vi "Set_Osc_Conf.vi"(0 "VISA resource name":refnum<visa-resource-name>="Oscilloscope", 1 "Amplitude IN":dbl=0.25, 2 "Trigger Level IN":dbl=0.025, 3 "Pulse Width in seconds IN":dbl=2.5e-09, 5 "error in (no error)":errorcluster, 6 "Channel 1":bool=TRUE, 7 "Channel 3":bool=TRUE, 8 "Channel 2":bool, 9 "Channel 4":bool=TRUE) -> (14 "VISA resource name out":refnum<visa-resource-name>="Oscilloscope", 19 "error out":errorcluster)   [LabVIEW 2012]
uses:
  C/Program Files/National Instruments/LabVIEW 2012/instr.lib/Agilent 8000 Series/Public/Configure/Configure Trigger (Edge).vi
  C/Program Files/National Instruments/LabVIEW 2012/instr.lib/Agilent 8000 Series/Agilent 8000 Series.lvlib
panel:
  in  "Channel 4":i32(ring)=4 items=["Channel 1"=1, "Channel 2"=2, "Channel 3"=3, "Channel 4"=4]
  in  "Vertical Coupling 4":i32(ring)=1 items=["AC", "DC"]
  in  "Probe Attenuation 4":dbl=1.0
  in  "Vertical Range Scaler 4":dbl=1.0
  in  "Vertical Offset 4":dbl
  in  "Input Impedance 4":u32(ring) items=["50 ohms", "1 Mohms"]
  in  "Channel 3":i32(ring)=3 items=["Channel 1"=1, "Channel 2"=2, "Channel 3"=3, "Channel 4"=4]
  in  "Vertical Coupling 3":i32(ring)=1 items=["AC", "DC"]
  in  "Probe Attenuation 3":dbl=1.0
  in  "Vertical Range Scaler 3":dbl=1.0
  in  "Vertical Offset 3":dbl
  in  "Input Impedance 3":u32(ring) items=["50 ohms", "1 Mohms"]
  in  "Channel 2":i32(ring)=2 items=["Channel 1"=1, "Channel 2"=2, "Channel 3"=3, "Channel 4"=4]
  in  "Vertical Coupling 2":i32(ring)=1 items=["AC", "DC"]
  in  "Probe Attenuation 2":dbl=1.0
  in  "Vertical Range Scaler 2":dbl=2.0
  in  "Vertical Offset 2":dbl
  in  "Input Impedance 2":u32(ring) items=["50 ohms", "1 Mohms"]
  in  "Trigger Coupling":u16(ring)=1 items=["AC", "DC", "Low Freq Reject", "High Freq Reject"]
  in  "Trigger Slope":u16(ring)=1 items=["Positive", "Negative"]
  in  "Trigger Source":i32(ring)=1 items=["Channel 1"=1, "Channel 2"=2, "Channel 3"=3, "Channel 4"=4, "Digital 0"=13, "Digital 1"=14, "Digital 2"=15, "Digital 3"=16, "Digital 4"=17, "Digital 5"=18, "Digital 6"=19, "Digital 7"=20, "Digital 8"=21, "Digital 9"=22, "Digital 10"=23, "Digital 11"=24, "Digital 12"=25, "Digital 13"=26, "Digital 14"=27, "Digital 15"=28, "Aux"=29, "Line"=30]
  in  "Timebase Scaler":dbl=20.0
  in  "Position 1":dbl
  in  "Record Length":i32=5000
  in  "Input Impedance 1":u32(ring) items=["50 ohms", "1 Mohms"]
  in  "Vertical Offset 1":dbl
  in  "Vertical Range Scaler 1":dbl=2.0
  in  "Probe Attenuation 1":dbl=1.0
  in  "Vertical Coupling 1":i32(ring)=1 items=["AC", "DC"]
  in  "Channel 1":i32(ring)=1 items=["Channel 1"=1, "Channel 2"=2, "Channel 3"=3, "Channel 4"=4]
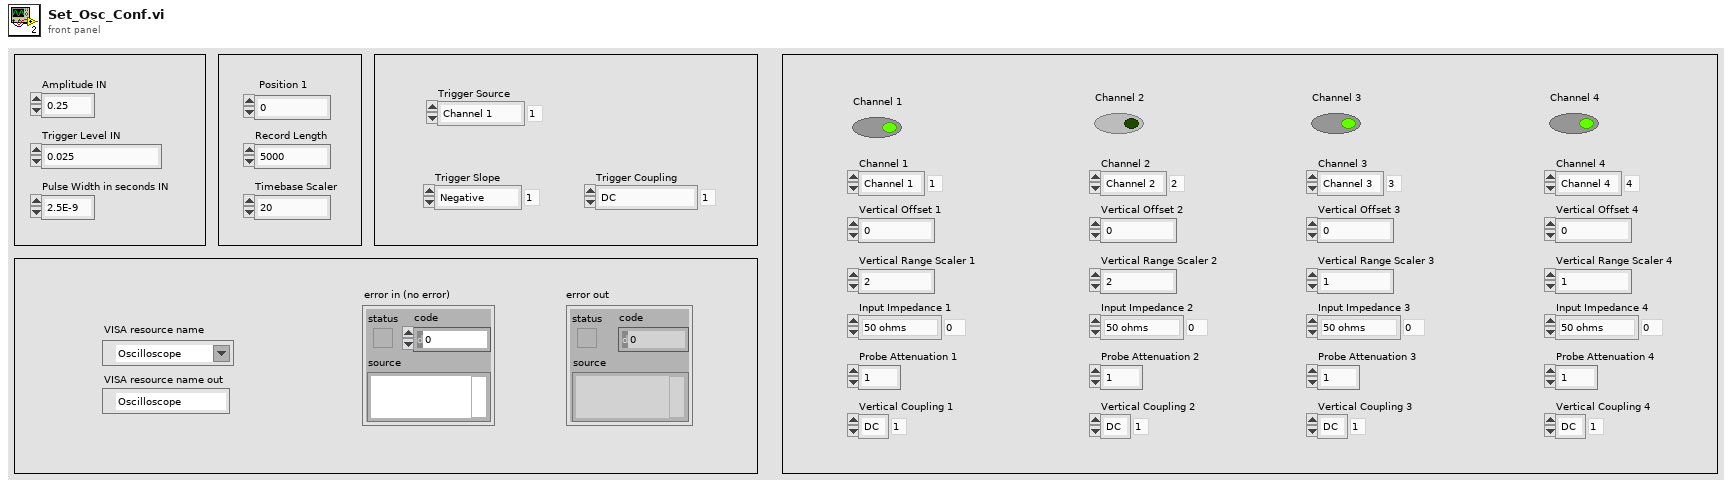
[diagram p1: front panel]
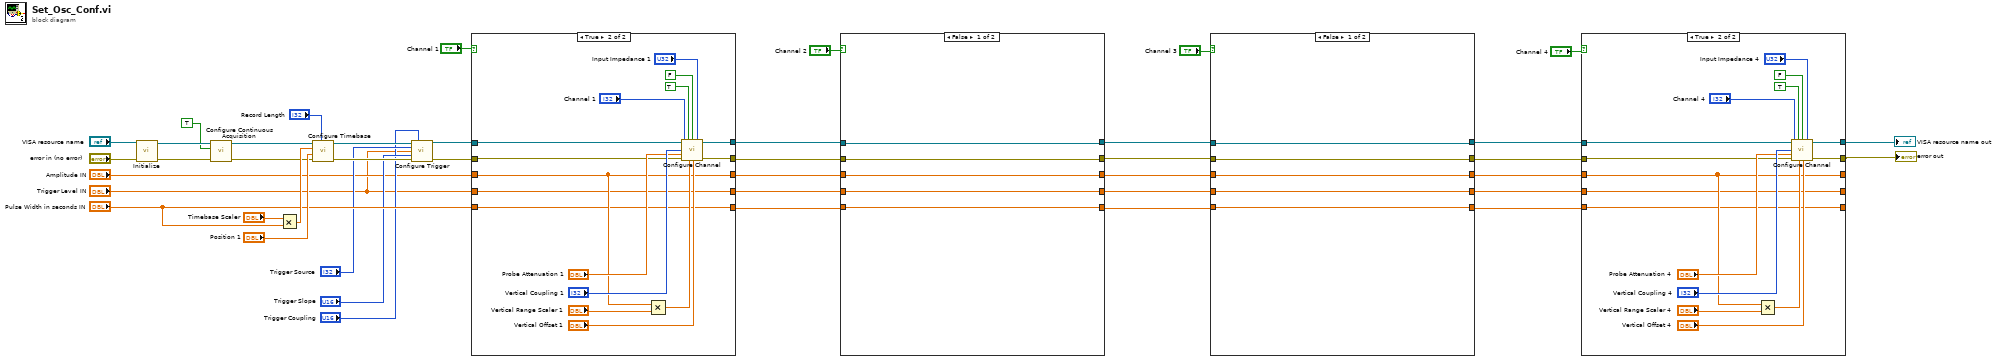
[diagram p0: block diagram]
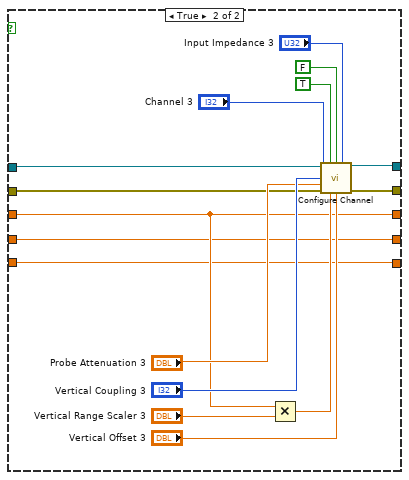
[diagram p3: hidden frame]
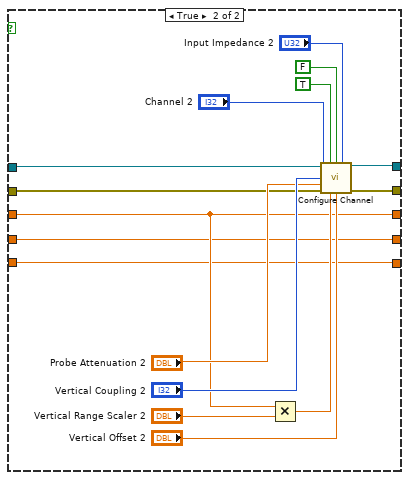
[diagram p4: hidden frame]
diagram:
  n1 = call <instrlib>:"Initialize.vi"("error in (no error)"="error in (no error)", "VISA resource name"="VISA resource name") -> ("error out"=w2:errorcluster, "VISA resource name out"=w5:refnum<visa-resource-name>)  [unwired: 8 in]
  n2 = call "Configure Continuous Acquisition.vi"("error in (no error)"=w2, "Enable Continuous Acquisition Mode (T:Enable)"=TRUE, "VISA resource name"=w5) -> ("error out"=w3:errorcluster, "VISA resource name out"=w4:refnum<visa-resource-name>)  [unwired: 7 in]
  n3 = Multiply(x="Timebase Scaler", y="Pulse Width in seconds IN") -> (x*y=w37:dbl)
  n4 = call <instrlib>:"Configure Timebase.vi"("Record Length (1000)"="Record Length", "error in (no error)"=w3, "Position (0.0 s)"="Position 1", "Timebase (0.005 s)"=w37, "VISA resource name"=w4) -> ("error out"=w32:errorcluster, "VISA resource name out"=w34:refnum<visa-resource-name>)  [unwired: 5 in]
  n5 = call-poly "Configure Trigger.vi"("VISA resource name"=w34, "Trigger Coupling (1 : DC)"="Trigger Coupling", "Trigger Source (1: Channel 1)"="Trigger Source", "Trigger Level (0.0 V)"="Trigger Level IN", "Trigger Slope (0: Positive)"="Trigger Slope", "error in (no error)"=w32) -> ("VISA resource name out"=w33:refnum<visa-resource-name>, "error out"=w31:errorcluster)  [unwired: 8 in]
  n6 = case shown="True" "Channel 1" {
    tunnel: w31 -> [w46 w51]
    tunnel: w33 -> [w47 w52]
    tunnel: "Amplitude IN" -> [w45 w50]
    tunnel: [w47 w54] -> w26
    tunnel: [w46 w53] -> w25
    tunnel: "Trigger Level IN" -> [w44 w49]
    tunnel: [w45 w50] -> w24
    tunnel: [w44 w49] -> w23
    tunnel: "Pulse Width in seconds IN" -> [w43 w48]
    tunnel: [w43 w48] -> w22
    frame False {
    }
    frame True {
      n7 = Multiply(x=w50, y="Vertical Range Scaler 1") -> (x*y=w58:dbl)
      n8 = call "Configure Channel.vi"("VISA resource name"=w52, "Enable Channel (Enable)"=TRUE, "BW Limit 20MHz (Disable)"=FALSE, "Input Impedance (1: 1 Mohms)"="Input Impedance 1", "Channel (1: Channel 1)"="Channel 1", "Vertical Coupling (1: DC)"="Vertical Coupling 1", "Probe Attenuation (1.0)"="Probe Attenuation 1", "error in (no error)"=w51, "Vertical Range (2.0 V)"=w58, "Vertical Offset (0.0 V)"="Vertical Offset 1") -> ("VISA resource name out"=w54:refnum<visa-resource-name>, "error out"=w53:errorcluster)  [unwired: 4 in]
    }
  }
  n9 = case shown="False" "Channel 2" {
    tunnel: w25 -> [w67 w72]
    tunnel: w26 -> [w68 w73]
    tunnel: w24 -> [w66 w71]
    tunnel: [w68 w75] -> w20
    tunnel: [w67 w74] -> w19
    tunnel: w23 -> [w65 w70]
    tunnel: [w66 w71] -> w18
    tunnel: [w65 w70] -> w17
    tunnel: w22 -> [w64 w69]
    tunnel: [w64 w69] -> w16
    frame False {
    }
    frame True {
      n10 = Multiply(x=w71, y="Vertical Range Scaler 2") -> (x*y=w79:dbl)
      n11 = call "Configure Channel.vi"("VISA resource name"=w73, "Enable Channel (Enable)"=TRUE, "BW Limit 20MHz (Disable)"=FALSE, "Input Impedance (1: 1 Mohms)"="Input Impedance 2", "Channel (1: Channel 1)"="Channel 2", "Vertical Coupling (1: DC)"="Vertical Coupling 2", "Probe Attenuation (1.0)"="Probe Attenuation 2", "error in (no error)"=w72, "Vertical Range (2.0 V)"=w79, "Vertical Offset (0.0 V)"="Vertical Offset 2") -> ("VISA resource name out"=w75:refnum<visa-resource-name>, "error out"=w74:errorcluster)  [unwired: 4 in]
    }
  }
  n12 = case shown="False" "Channel 3" {
    tunnel: w19 -> [w88 w93]
    tunnel: w20 -> [w89 w94]
    tunnel: w18 -> [w87 w92]
    tunnel: [w89 w96] -> w14
    tunnel: [w88 w95] -> w13
    tunnel: w17 -> [w86 w91]
    tunnel: [w87 w92] -> w12
    tunnel: [w86 w91] -> w11
    tunnel: w16 -> [w85 w90]
    tunnel: [w85 w90] -> w10
    frame False {
    }
    frame True {
      n13 = Multiply(x=w92, y="Vertical Range Scaler 3") -> (x*y=w100:dbl)
      n14 = call "Configure Channel.vi"("VISA resource name"=w94, "Enable Channel (Enable)"=TRUE, "BW Limit 20MHz (Disable)"=FALSE, "Input Impedance (1: 1 Mohms)"="Input Impedance 3", "Channel (1: Channel 1)"="Channel 3", "Vertical Coupling (1: DC)"="Vertical Coupling 3", "Probe Attenuation (1.0)"="Probe Attenuation 3", "error in (no error)"=w93, "Vertical Range (2.0 V)"=w100, "Vertical Offset (0.0 V)"="Vertical Offset 3") -> ("VISA resource name out"=w96:refnum<visa-resource-name>, "error out"=w95:errorcluster)  [unwired: 4 in]
    }
  }
  n15 = case shown="True" "Channel 4" {
    tunnel: w13 -> [w109 w114]
    tunnel: w14 -> [w110 w115]
    tunnel: w12 -> [w108 w113]
    tunnel: [w110 w117] -> w9
    tunnel: [w109 w116] -> w7
    tunnel: w11 -> [w107 w112]
    tunnel: [w108 w113] -> _
    tunnel: [w107 w112] -> _
    tunnel: w10 -> [w106 w111]
    tunnel: [w106 w111] -> _
    frame False {
    }
    frame True {
      n16 = Multiply(x=w113, y="Vertical Range Scaler 4") -> (x*y=w121:dbl)
      n17 = call "Configure Channel.vi"("VISA resource name"=w115, "Enable Channel (Enable)"=TRUE, "BW Limit 20MHz (Disable)"=FALSE, "Input Impedance (1: 1 Mohms)"="Input Impedance 4", "Channel (1: Channel 1)"="Channel 4", "Vertical Coupling (1: DC)"="Vertical Coupling 4", "Probe Attenuation (1.0)"="Probe Attenuation 4", "error in (no error)"=w114, "Vertical Range (2.0 V)"=w121, "Vertical Offset (0.0 V)"="Vertical Offset 4") -> ("VISA resource name out"=w117:refnum<visa-resource-name>, "error out"=w116:errorcluster)  [unwired: 4 in]
    }
  }
  "VISA resource name out" <- w9
  "error out" <- w7
